vi "Basic.vi"() -> ()   [LabVIEW 2020]
panel:
  in  "stop":bool
  out "x+y":dbl
  in  "Number 2":dbl
  in  "Boolean":bool
  in  "Number":dbl
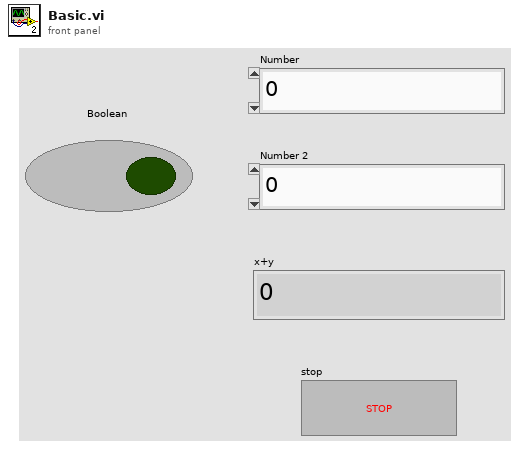
[diagram p1: front panel]
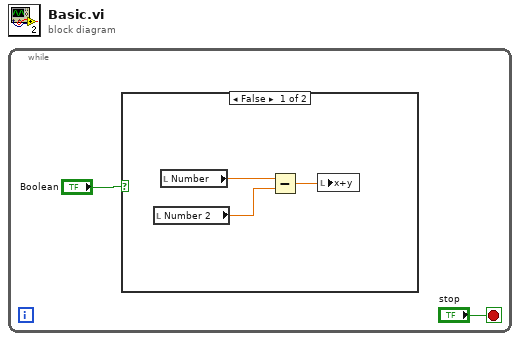
[diagram p0: block diagram]
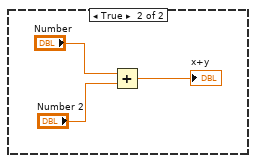
[diagram p2: hidden frame]
diagram:
  n1 = while {
    stop <- "stop" stop-if-true
    n2 = case shown="False" "Boolean" {
      frame False {
        n3 = local read "Number 2"() -> (w4:dbl)
        n4 = local read "Number"() -> (w5:dbl)
        n5 = Subtract(x=w5, y=w4) -> (x-y=w3:dbl)
        n6 = local write "x+y"(w3) -> ()
      }
      frame True {
        n7 = Add(x="Number", y="Number 2") -> (x+y=→"x+y":dbl)
      }
    }
  }
